vi "Assisted Turning.vi"(1 "Left":bool=TRUE, 2 "Current Value":dbl format="%#_13g", 3 "Right":bool, 4 "Turn Amount":dbl format="%#_13g") -> (0 "New Value":dbl format="%#_13g")   [LabVIEW 2016]
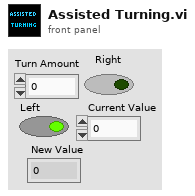
[diagram p1: front panel]
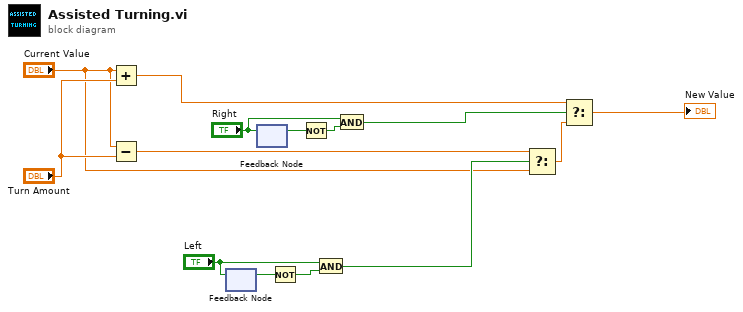
[diagram p0: block diagram]
diagram:
  n1 = Add(x="Current Value", y="Turn Amount") -> (x+y=w2:dbl)
  n2 = Subtract(x="Current Value", y="Turn Amount") -> (x-y=w3:dbl)
  n3 = feedback-in #1("Left") -> ()
  n4 = feedback #1() -> (w13:bool)  [unwired: 1 in]
  n5 = feedback-in #2("Right") -> ()
  n6 = feedback #2() -> (w9:bool)  [unwired: 1 in]
  n7 = Not(x=w13) -> (.not. x?=w12:bool)
  n8 = Not(x=w9) -> (.not. x?=w10:bool)
  n9 = And(x="Left", y=w12) -> (x .and. y?=w7:bool)
  n10 = And(x="Right", y=w10) -> (x .and. y?=w6:bool)
  n11 = Select(t=w3, s=w7, f="Current Value") -> (s? t:f=w8:dbl)
  n12 = Select(t=w2, s=w6, f=w8) -> (s? t:f=→"New Value":dbl)
